vi "GV_SetGraph.vi"(8 "error in (no error)":errorcluster, 11 "Gviewer in":refnum<class "Gviewer.lvclass">) -> (0 "error out":errorcluster, 3 "Gviewer out":refnum<class "Gviewer.lvclass">)   [LabVIEW 2014, in "Gviewer.lvclass"]
doc: "Set the Size and Position of the Graph"
uses:
  Gviewer.lvclass
  <vilib>/Utility/miscctls.llb/LVPositionTypeDef.ctl
  <vilib>/Utility/miscctls.llb/LVBoundsTypeDef.ctl
  Gviewer.lvclass/Gviewer.ctl
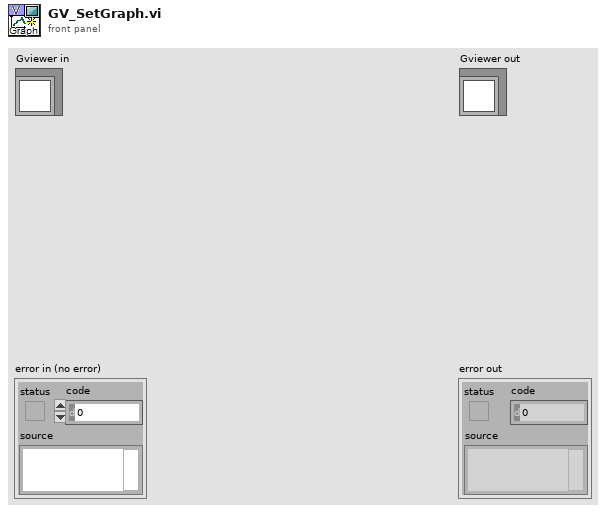
[diagram p1: front panel]
types:
  T1 = typedef "LVBoundsTypeDef.ctl" = cluster{"Width":u32, "Height":u32}
  T2 = typedef "LVPositionTypeDef.ctl" = cluster{"Left":i32, "Top":i32}
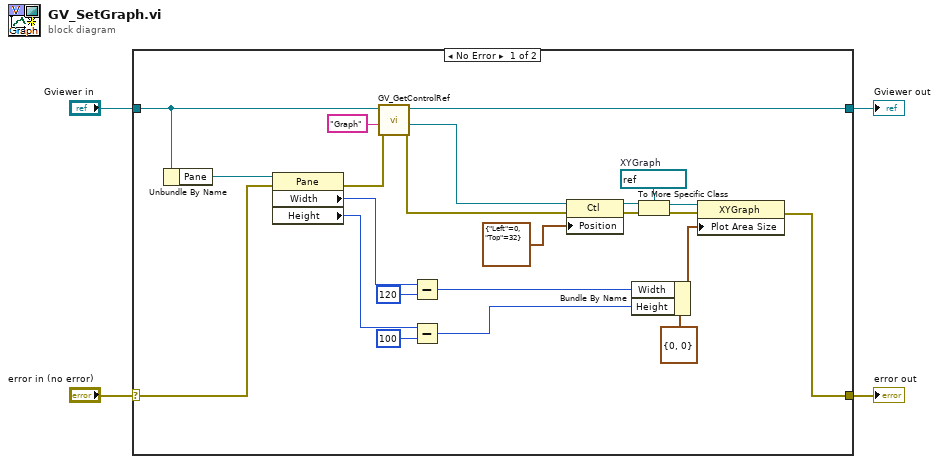
[diagram p0: block diagram]
diagram:
  n1 = case shown="No Error" "error in (no error)" {
    selector: "error in (no error)" -> [w13 w29]
    tunnel: [w9 w29] -> w3
    tunnel: [w12 w28] -> w1
    tunnel: "Gviewer in" -> [w11 w28]
    frame No Error {
      w22 = refnum<vi> refnum  # XYGraph
      n2 = Unbundle By Name(w11) -> ("Pane"=w10:refnum<vi>)
      n3 = property class="Pane"(reference=w10, error in=w13) -> (error out=w17:errorcluster, "Width"=w16:u32, "Height"=w8:u32)  [unwired: 1 out]
      n4 = call "GV_GetControlRef.vi"("error in (no error)"=w17, "CNT name"="Graph", "Gviewer in"=w11) -> ("error out"=w25:errorcluster, "Reference"=w26:refnum<vi>, "Gviewer out"=w12:refnum<class "Gviewer.lvclass">)  [unwired: 6 in]
      n5 = Subtract(x=w16, y=u32 120) -> (x-y=w14:u32)
      n6 = Subtract(x=w8, y=u32 100) -> (x-y=w6:u32)
      n7 = property class="Ctl"(reference=w26, error in=w25, "Position"=T2 {"Left"=0, "Top"=32}) -> (reference out=w23:refnum<vi>, error out=w21:errorcluster)
      n8 = Bundle By Name(cluster=T1 {"Width"=0, "Height"=0} ("Draw Area Size"), "Width"=w14, "Height"=w6) -> (w5:T1)
      n9 = To More Specific Class(target class=w22, reference=w23, error in=w21) -> (specific class reference=w20:refnum<vi>, error out=w19:errorcluster)
      n10 = property class="XYGraph"(reference=w20, error in=w19, "Plot Area Size"=w5) -> (error out=w9:errorcluster)  [unwired: 1 out]
    }
    frame Error {
    }
  }
  "error out" <- w3
  "Gviewer out" <- w1
